vi "final project.vi"() -> ()   [LabVIEW 2014]
panel:
  out "using time(s)":dbl
  out "score":u8
  in  "plane":T1
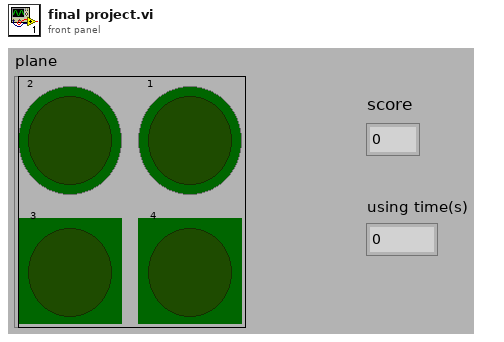
[diagram p1: front panel]
types:
  T1 = cluster{"2":bool, "1 ":bool, " 3":bool, " 4":bool}
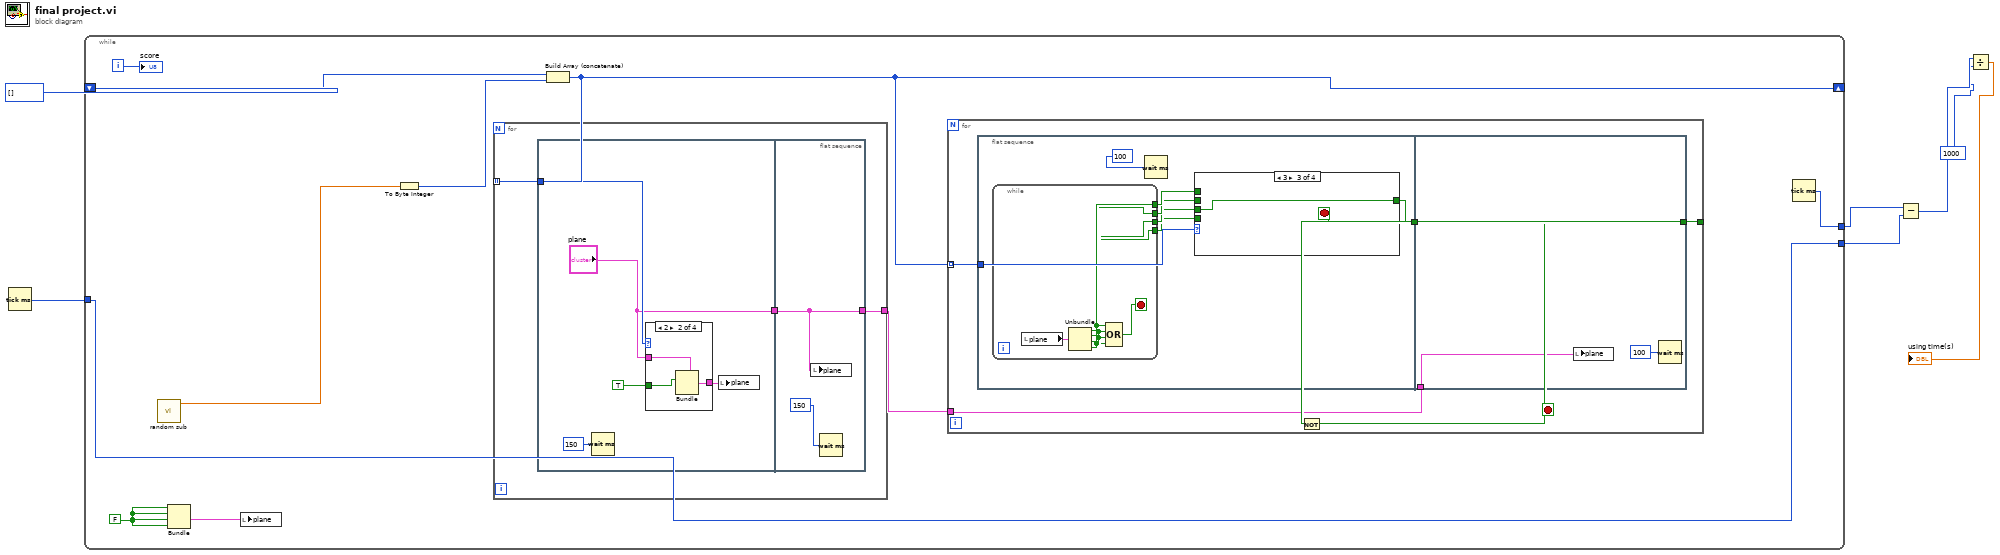
[diagram p0: block diagram]
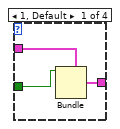
[diagram p5: hidden frame]
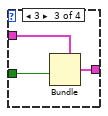
[diagram p6: hidden frame]
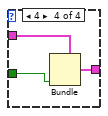
[diagram p7: hidden frame]
diagram:
  n1 = Tick Count (ms)() -> (millisecond timer value=w6:u32)
  n2 = while {
    shift-right: [w15] -> _
    shift-left: i32[] [] -> [w17]
    tunnel: w6 -> [w10]
    tunnel: [w10] -> w5
    tunnel: [w8] -> w1
    i -> [w11]
    stop <- w16 stop-if-true
    w13 = FALSE
    n3 = call "random sub.vi"() -> ("Numeric"=w9:dbl)  [unwired: 11 in]
    n4 = Bundle(w13, w13, w13, w13) -> (w12:cluster{bool, bool, bool, bool})  [unwired: 1 in]
    n5 = local write "plane"(w12) -> ()
    n6 = To Byte Integer(number=w9) -> (8bit integer=w18:i8)
    n7 = Build Array (concatenate)(w17, w18) -> (w15:i32[])
    n8 = for {
      tunnel: w15 -> [w46] mode=indexing
      tunnel: [w44] -> w14
      n9 = flat-sequence {
        tunnel: w46 -> [w51]
        tunnel: ["plane"] -> w45
        tunnel: w45 -> [w64]
        tunnel: [w64] -> w44
        frame #0 {
          n10 = Wait (ms)(milliseconds to wait=u32 150) -> ()  [unwired: 1 out]
          n11 = case shown="2" w51 {
            tunnel: "plane" -> [w54 w57 w59 w63]
            tunnel: TRUE -> [w53 w56 w60 w62]
            tunnel: [w52 w55 w58 w61] -> w48
            frame 1, Default {
              n12 = Bundle(cluster=w54, "2"=w53) -> (w52:T1)  [unwired: 3 in]
            }
            frame 2 {
              n13 = Bundle(cluster=w57, "1"=w56) -> (w55:T1)  [unwired: 3 in]
            }
            frame 3 {
              n14 = Bundle(cluster=w59, "3"=w60) -> (w58:T1)  [unwired: 3 in]
            }
            frame 4 {
              n15 = Bundle(cluster=w63, "4"=w62) -> (w61:T1)  [unwired: 3 in]
            }
          }
          n16 = local write "plane"(w48) -> ()
        }
        frame #1 {
          n17 = local write "plane"(w64) -> ()
          n18 = Wait (ms)(milliseconds to wait=u32 150) -> ()  [unwired: 1 out]
        }
      }
    }
    n19 = for {
      tunnel: w15 -> [w23] mode=indexing
      tunnel: [w20] -> w16
      tunnel: w14 -> [w19]
      stop <- w20 stop-if-true
      n20 = flat-sequence {
        tunnel: w23 -> [w30]
        tunnel: [w25] -> w22
        tunnel: w22 -> [w41]
        tunnel: w19 -> [w43]
        tunnel: [w41] -> w21
        frame #0 {
          n21 = while {
            tunnel: [w38] -> w29
            tunnel: [w37] -> w28
            tunnel: [w36] -> w27
            tunnel: [w35] -> w26
            stop <- w39 stop-if-true
            n22 = local read "plane"() -> (w40:T1)
            n23 = Unbundle(w40) -> ("2"=w38:bool, "1"=w37:bool, "3"=w36:bool, "4"=w35:bool)
            n24 = Compound Arithmetic op=OR(w38, w37, w36, w35) -> (w39:bool)
          }
          n25 = Wait (ms)(milliseconds to wait=u32 100) -> ()  [unwired: 1 out]
          n26 = case shown="3" w30 {
            tunnel: [w31 w32 w33 w34] -> w25
            tunnel: w29 -> [w31 _ _ _]
            tunnel: w28 -> [_ w32 _ _]
            tunnel: w27 -> [_ _ w33 _]
            tunnel: w26 -> [_ _ _ w34]
            frame 1, Default {
            }
            frame 2 {
            }
            frame 3 {
            }
            frame 4 {
            }
          }
        }
        frame #1 {
          n27 = local write "plane"(w43) -> ()
          n28 = Wait (ms)(milliseconds to wait=u32 100) -> ()  [unwired: 1 out]
        }
      }
      n29 = Not(x=w21) -> (.not. x?=w20:bool)
    }
    n30 = Tick Count (ms)() -> (millisecond timer value=w8:u32)
    "score" <- w11
  }
  n31 = Subtract(x=w1, y=w5) -> (x-y=w4:u32)
  n32 = Divide(x=w4, y=1000) -> (x/y=→"using time(s)":dbl)
